vi "Get Font.vi"(8 "error in":errorcluster, 10 "Font":T1={"Bold"=enum."Bold true", "Italic"=enum."Unchanged", "Underline"=enum."none", "Color"=0, "Size"=-1.0, "Name"=""}, 11 "SpreadsheetDoc in":refnum<k24>) -> (0 "error out":errorcluster, 1 "FontId":i32, 2 "Font":refnum<k24>, 3 "SpreadsheetDoc out":refnum<k24>)   [LabVIEW 2021, in "Open Xml.lvlib"]
uses:
  Open Xml.lvlib
  D:/git/Open-Xml-LabVIEW/dll/DocumentFormat.OpenXml.Framework.dll
  dll/DocumentFormat.OpenXml.Framework.dll
  D:/git/Open-Xml-LabVIEW/dll/DocumentFormat.OpenXml.dll
  dll/DocumentFormat.OpenXml.dll
  Font.ctl
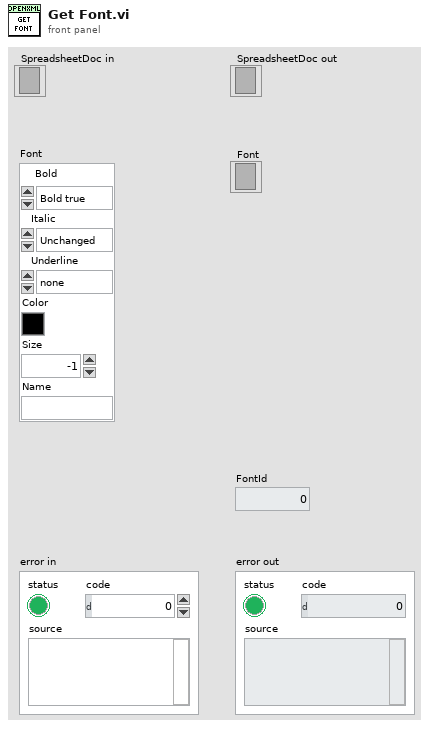
[diagram p1: front panel]
types:
  T1 = typedef "Open Xml.lvlib/Font.ctl" = cluster{"Bold":enum16{"Bold true", "Bold false", "Unchanged"}, "Italic":enum16{"Italic true", "Italic false", "Unchanged"}, "Underline":enum16{"single", "double", "singleAccounting", "doubleAccounting", "none", "Unchanged"}, "Color":u32, "Size":dbl, "Name":string}
  T2 = enum16{"single", "double", "singleAccounting", "doubleAccounting", "none", "Unchanged"}
  T3 = enum16{"Italic true", "Italic false", "Unchanged"}
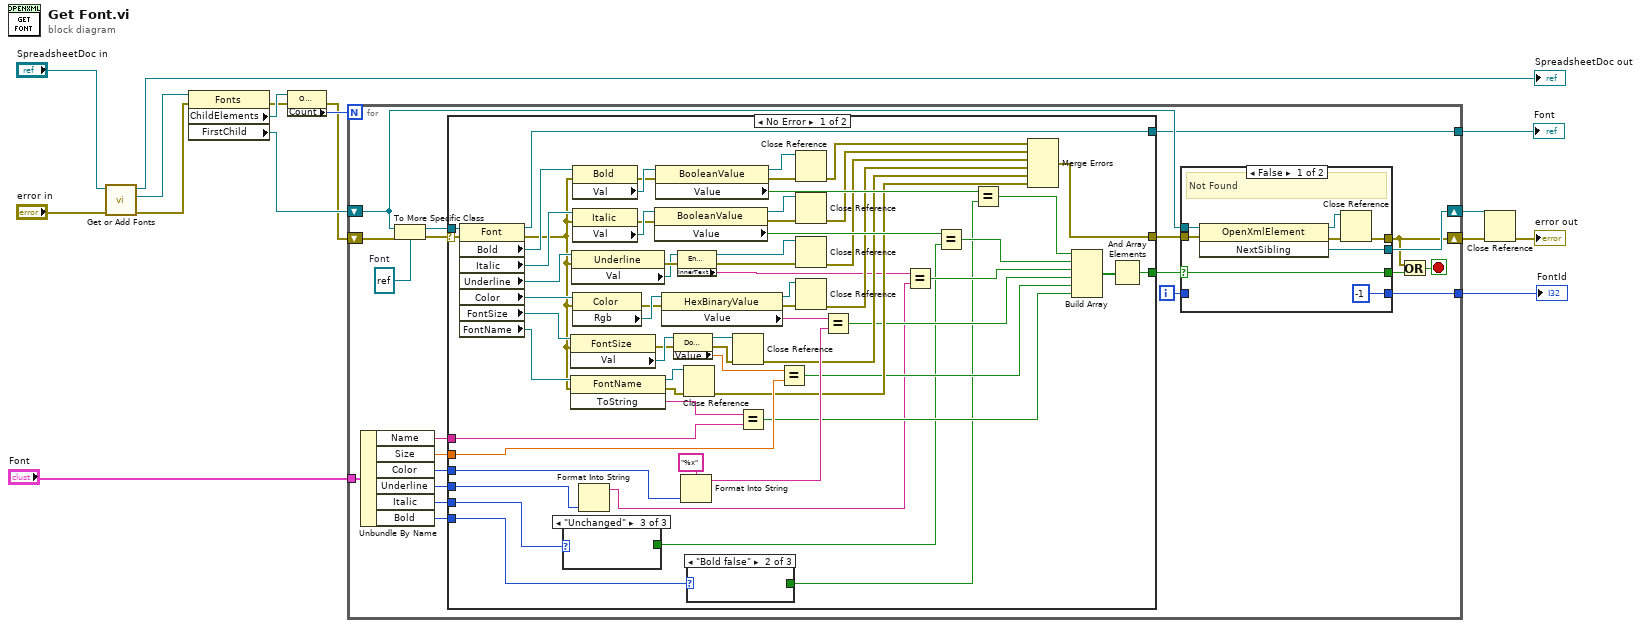
[diagram p0: block diagram]
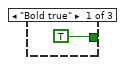
[diagram p2: hidden frame]
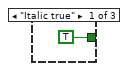
[diagram p4: hidden frame]
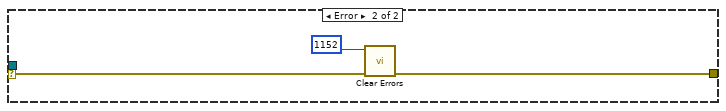
[diagram p6: hidden frame]
diagram:
  n1 = call "Get or Add Fonts.vi"("error in"="error in", "SpreadsheetDoc in"="SpreadsheetDoc in") -> ("error out"=w10:errorcluster, "Fonts"=w13:refnum<k24>, "SpreadsheetDoc out"=→"SpreadsheetDoc out":refnum<k24>)  [unwired: 7 in]
  n2 = property class="Fonts"(reference=w13, error in=w10) -> (error out=w9:errorcluster, "ChildElements"=w12:refnum<k24>, "FirstChild"=w8:refnum<k24>)  [unwired: 1 out]
  n3 = property class="OpenXmlElementList"(reference=w12, error in=w9) -> (error out=w7:errorcluster, "Count"=w11:i32)  [unwired: 1 out]
  n4 = for {
    N: w11 -> [_]
    shift-right: [w22] -> w3
    shift-left: w8 -> [w26]
    shift-right: [w21] -> w6
    shift-left: w7 -> [w36]
    tunnel: "Font" -> [w33]
    tunnel: [w23] -> w5
    tunnel: [w17] -> w1
    i -> [w18]
    stop <- w24 stop-if-true
    w35 = refnum<k24> refnum  # Font
    n5 = Unbundle By Name(w33) -> ("Name"=w32:string, "Size"=w31:dbl, "Color"=w30:u32, "Underline"=w29:T2, "Italic"=w28:T3, "Bold"=w27:enum16{"Bold true", "Bold false", "Unchanged"})
    n6 = To More Specific Class(target class=w35, reference=w26, error in=w36) -> (specific class reference=w37:refnum<k24>, error out=w34:errorcluster)
    n7 = case shown="No Error" w34 {
      selector: w34 -> [w100 w106]
      tunnel: w37 -> [w101 _]
      tunnel: w32 -> [w88 _]
      tunnel: w31 -> [w86 _]
      tunnel: w30 -> [w85 _]
      tunnel: w29 -> [w43 _]
      tunnel: w28 -> [w41 _]
      tunnel: w27 -> [w39 _]
      tunnel: [w48 w105] -> w25
      tunnel: [w47 _] -> w20
      tunnel: [w46 _] -> w23
      frame No Error {
        n8 = property class="Font"(reference=w101, error in=w100) -> (reference out=w46:refnum<k24>, error out=w90:errorcluster, "Bold"=w99:refnum<k24>, "Italic"=w98:refnum<k24>, "Underline"=w97:refnum<k24>, "Color"=w96:refnum<k24>, "FontSize"=w95:refnum<k24>, "FontName"=w94:refnum<k24>)
        n9 = case shown="\"Unchanged\"" w41 {
          tunnel: [TRUE _ _] -> w40
          frame "Italic true" {
          }
          frame "Italic false" {
          }
          frame "Unchanged" {
          }
        }
        n10 = property class="FontSize"(reference=w95, error in=w90) -> (error out=w75:errorcluster, "Val"=w91:refnum<k24>)  [unwired: 1 out]
        n11 = invoke class="FontName" method="ToString"(reference=w94, error in=w90) -> (reference out=w63:refnum<k24>, error out=w62:errorcluster, "ToString"=w89:string)  [unwired: 1 in]
        n12 = property class="Underline"(reference=w97, error in=w90) -> (error out=w78:errorcluster, "Val"=w77:refnum<k24>)  [unwired: 1 out]
        n13 = property class="Bold"(reference=w99, error in=w90) -> (error out=w81:errorcluster, "Val"=w82:refnum<k24>)  [unwired: 1 out]
        n14 = property class="Italic"(reference=w98, error in=w90) -> (error out=w79:errorcluster, "Val"=w80:refnum<k24>)  [unwired: 1 out]
        n15 = property class="Color"(reference=w96, error in=w90) -> (error out=w76:errorcluster, "Rgb"=w93:refnum<k24>)  [unwired: 1 out]
        n16 = Format Into String(w43) -> (resulting string=w42:string)  [unwired: 3 in, 1 out]
        n17 = property class="BooleanValue"(reference=w80, error in=w79) -> (reference out=w71:refnum<k24>, error out=w70:errorcluster, "Value"=w73:bool)
        n18 = property class="BooleanValue"(reference=w82, error in=w81) -> (reference out=w72:refnum<k24>, error out=w69:errorcluster, "Value"=w74:bool)
        n19 = property class="HexBinaryValue"(reference=w93, error in=w76) -> (reference out=w66:refnum<k24>, error out=w67:errorcluster, "Value"=w92:string)
        n20 = property class="DoubleValue"(reference=w91, error in=w75) -> (reference out=w65:refnum<k24>, error out=w64:errorcluster, "Value"=w87:dbl)
        n21 = property class="EnumValue`1[[DocumentFormat.Ope"(reference=w77, error in=w78) -> (reference out=w68:refnum<k24>, error out=w45:errorcluster, "InnerText"=w44:string)
        n22 = Format Into String(format string="%x", w85) -> (resulting string=w83:string)  [unwired: 2 in, 1 out]
        n23 = Close Reference(reference=w63, error in (no error)=w62) -> (error out=w53:errorcluster)
        n24 = case shown="\"Bold false\"" w39 {
          tunnel: [TRUE _ _] -> w38
          frame "Bold true" {
          }
          frame "Bold false" {
          }
          frame "Unchanged", Default {
          }
        }
        n25 = Close Reference(reference=w65, error in (no error)=w64) -> (error out=w54:errorcluster)
        n26 = Equal?(x=w89, y=w88) -> (x = y?=w50:bool)
        n27 = Equal?(x=w87, y=w86) -> (x = y?=w51:bool)
        n28 = Close Reference(reference=w72, error in (no error)=w69) -> (error out=w61:errorcluster)
        n29 = Close Reference(reference=w71, error in (no error)=w70) -> (error out=w60:errorcluster)
        n30 = Close Reference(reference=w68, error in (no error)=w45) -> (error out=w56:errorcluster)
        n31 = Close Reference(reference=w66, error in (no error)=w67) -> (error out=w55:errorcluster)
        n32 = Equal?(x=w92, y=w83) -> (x = y?=w52:bool)
        n33 = Equal?(x=w44, y=w42) -> (x = y?=w57:bool)
        n34 = Equal?(x=w73, y=w40) -> (x = y?=w58:bool)
        n35 = Equal?(x=w74, y=w38) -> (x = y?=w59:bool)
        n36 = Merge Errors(w61, w60, w56, w55, w54, w53) -> (w48:errorcluster)
        n37 = Build Array(w59, w58, w57, w52, w51, w50) -> (w49:bool[])
        n38 = And Array Elements(Boolean array=w49) -> (logical AND=w47:bool)
      }
      frame Error {
        n39 = call <vilib>:"Clear Errors.vi"("error in (no error)"=w106, "specific error code to clear (0: all)"=1152) -> ("error out"=w105:errorcluster)  [unwired: 4 in, 1 out]
      }
    }
    n40 = case shown="False" w20 {
      selector: w20 -> [w108 w116]
      tunnel: w26 -> [w114 _]
      tunnel: w25 -> [w113 w117]
      tunnel: [w112 _] -> w22
      tunnel: [w109 w117] -> w21
      tunnel: [w108 w116] -> w19
      tunnel: w18 -> [_ w115]
      tunnel: [-1 w115] -> w17
      frame False {
        # "Not Found"
        n41 = invoke class="OpenXmlElement" method="NextSibling"(reference=w114, error in=w113) -> (reference out=w111:refnum<k24>, error out=w110:errorcluster, "NextSibling"=w112:refnum<k24>)  [unwired: 1 in]
        n42 = Close Reference(reference=w111, error in (no error)=w110) -> (error out=w109:errorcluster)
      }
      frame True {
        # "Found"
      }
    }
    n43 = Or(x=w21, y=w19) -> (x .or. y?=w24:bool)
  }
  "Font" <- w5
  "FontId" <- w1
  n44 = Close Reference(reference=w3, error in (no error)=w6) -> (error out=→"error out":errorcluster)
